vi "OAT LP Hilbert Transformer Kaiser Design.vi"(8 "A stop [dB]":dbl=72.0 format="%.2f", 9 "stopband":dbl=0.25 format="%.2f", 10 "passband":dbl=0.05 format="%.2f", 11 "fs":dbl=1.0 format="%.2f") -> (0 "error":i32, 2 "taps":i32, 3 "filter coefficients":dbl[](array[numeric]) format="%.2f")   [LabVIEW 2017, in "SoundVib_Resampling.lvlib"]
uses:
  <vilib>/addons/Sound and Vibration/Order Analysis/Resample Order Tracking/SoundVib_Resampling.lvlib
  <vilib>/Analysis/4window.llb/Kaiser-Bessel Window (DBL).vi
  <vilib>/Analysis/NI_AALPro.lvlib
panel:
  out "Waveform Graph":T1(graph)
  in  "debug?":bool
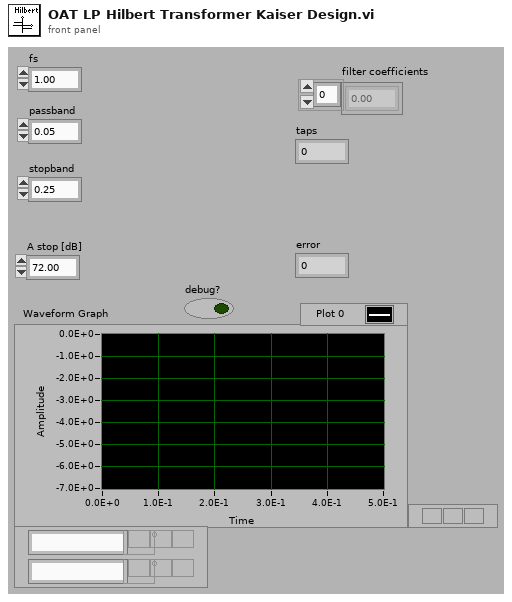
[diagram p1: front panel]
types:
  T1 = cluster{"Lower Freq":dbl, "df":dbl, "amplitude":dbl[]}
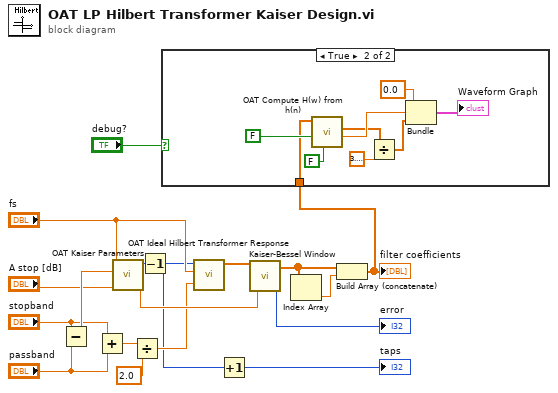
[diagram p0: block diagram]
diagram:
  n1 = Subtract(x="stopband", y="passband") -> (x-y=w13:dbl)
  n2 = Add(x="stopband", y="passband") -> (x+y=w4:dbl)
  n3 = call <vilib>:"OAT Kaiser Parameters.vi"("A stop [dB]"="A stop [dB]", "delta f"=w13, "fs"="fs") -> ("beta"=w10:dbl, "taps"=w9:i32)  [unwired: 7 in]
  n4 = Divide(x=w4, y=2.0) -> (x/y=w2:dbl)
  n5 = Decrement(x=w9) -> (x-1=w1:i32)
  n6 = call <vilib>:"OAT Ideal Hilbert Transformer Response.vi"("fc"=w2, "fs"="fs", "N"=w1) -> ("coef"=w5:dbl[])  [unwired: 8 in]
  n7 = Increment(x=w1) -> (x+1=→"taps":i32)
  n8 = call-poly <vilib>:"Kaiser-Bessel Window.vi"("beta"=w10, "X"=w5) -> ("error"=→"error":i32, "Windowed X"=w17:dbl[])
  n9 = Index Array(array=w17) -> (element=w16:dbl)  [unwired: 1 in]
  n10 = Build Array (concatenate)(w17, w16) -> (w12:dbl[])
  "filter coefficients" <- w12
  n11 = case shown="True" "debug?" {
    tunnel: w12 -> [_ w23]
    frame False {
    }
    frame True {
      n12 = call <vilib>:"OAT Compute H(w) from h(n).vi"("group delay?"=FALSE, "dB on?"=FALSE, "h[n]"=w23) -> ("df"=w26:dbl, "phase"=w20:dbl[])  [unwired: 6 in, 1 out]
      n13 = Divide(x=w20, y=3.141592653589793) -> (x/y=w19:dbl[])
      n14 = Bundle("Lower Freq"=0.0, "df"=w26, w19) -> (→"Waveform Graph":cluster{"Lower Freq":dbl, "df":dbl, dbl[]})  [unwired: 1 in]
    }
  }
